vi "ICR_Finish_Sequence.vi"(8 "error in (no error)":errorcluster, 11 "QMH ICR Cluster":T1) -> (0 "error out":errorcluster, 2 "Is Finished ?":bool, 3 "QMH ICR Cluster":T1)   [LabVIEW 2024]
doc: "This VI inits a waveform generation session for both HSDIO 6541 and AWG 5421. This is a basic example that shows how to setup the board in order to generate waveforms according to a script. \n\n1. Initialize for a generation session.\n2. Assign specified channels in Channel List for dynamic operation : all = \"\" (default)\n3. Sets the Idle State for when the generation has completed : NO !!\n4. Configure the Sample clock to use the onboard clock, and configure the clock rate.\n5. Set generation mode to Scripted.\n6. Configure the Script Trigger : change to Digital Edge if waiting for an external\n trigger, and link Rising Edge and source trigger commands.\n Use PFI0 with SMB wired to the board, or any PFIxx if connected to accessory."
uses:
  controls/QMH_ICR_Cluster.ctl
  controls/HARDWARE_Resources.ctl
  controls/PROCESSING_Inputs.ctl
  controls/LOOPS_Inputs.ctl
  controls/OPO_Inputs.ctl
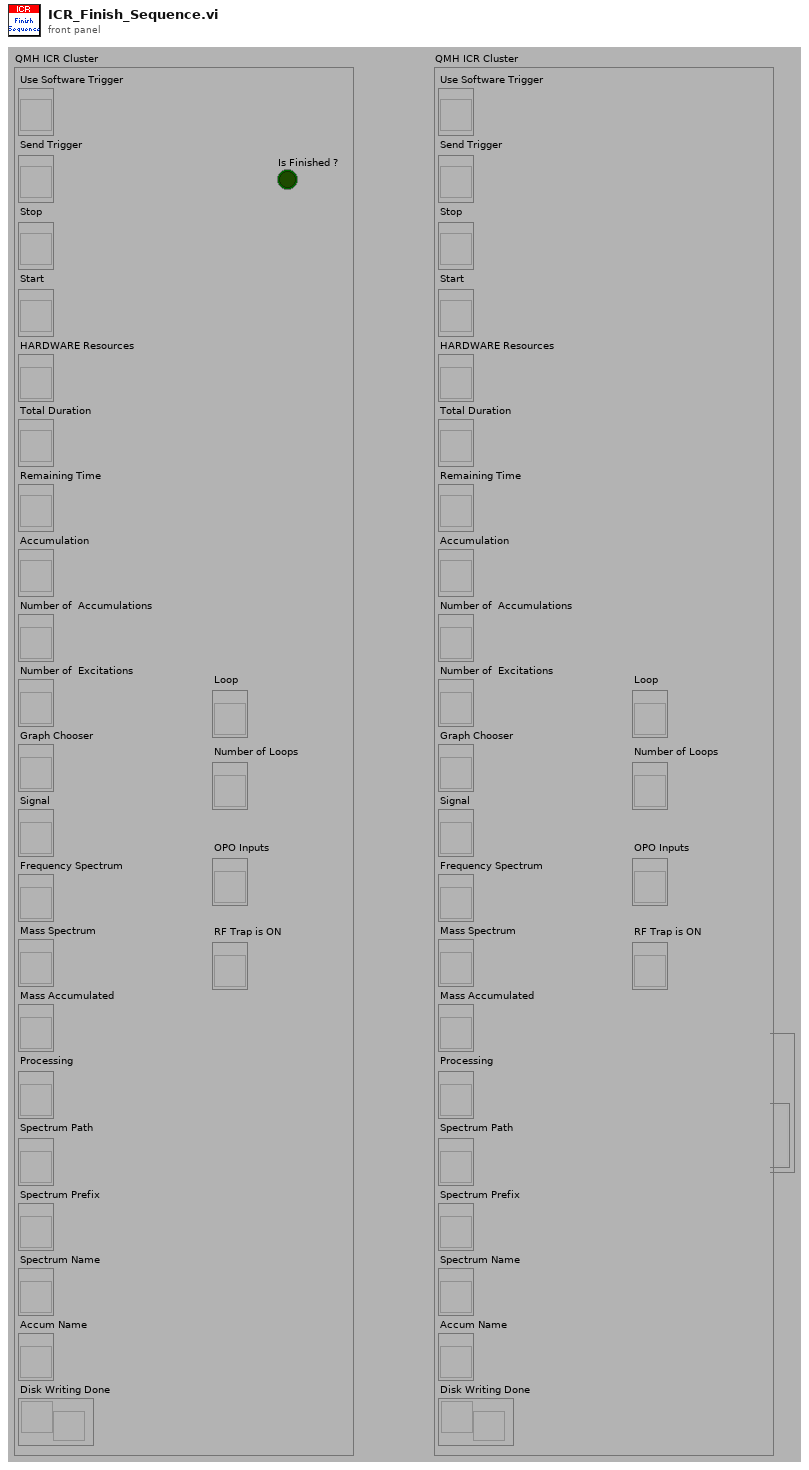
[diagram p1: front panel]
types:
  T1 = typedef "QMH_ICR_Cluster.ctl" = cluster{"Use Software Trigger":refnum<vi>, "Send Trigger":refnum<vi>, "Stop":refnum<vi>, "Start":refnum<vi>, "HARDWARE Resources":refnum<vi>, "Total Duration":refnum<vi>, "Remaining Time":refnum<vi>, "Accumulation":refnum<vi>, "Number of  Accumulations":refnum<vi>, "Number of  Excitations":refnum<vi>, "Graph Chooser":refnum<vi>, "Signal":refnum<vi>, "Frequency Spectrum":refnum<vi>, "Mass Spectrum":refnum<vi>, "Mass Accumulated":refnum<vi>, "Processing":refnum<vi>, "Spectrum Path":refnum<vi>, "Spectrum Prefix":refnum<vi>, "Spectrum Name":refnum<vi>, "Accum Name":refnum<vi>, "Disk Writing Done":refnum<notifier>, "Loop":refnum<vi>, "Number of Loops":refnum<vi>, "OPO Inputs":refnum<vi>, "RF Trap is ON":refnum<vi>}
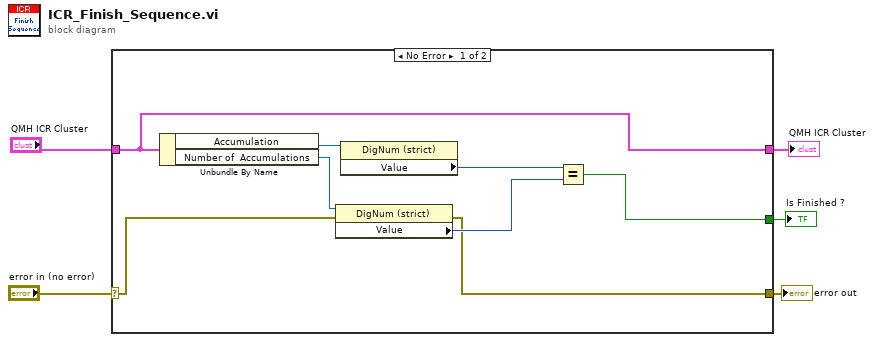
[diagram p0: block diagram]
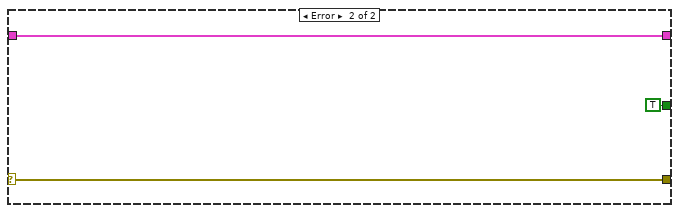
[diagram p2: hidden frame]
diagram:
  n1 = case shown="No Error" "error in (no error)" {
    selector: "error in (no error)" -> [w8 w16]
    tunnel: [w7 w16] -> w5
    tunnel: "QMH ICR Cluster" -> [w6 w15]
    tunnel: [w6 w15] -> w2
    tunnel: [w9 TRUE] -> w1
    frame No Error {
      n2 = Unbundle By Name(w6) -> ("Accumulation"=w12:refnum<vi>, "Number of  Accumulations"=w13:refnum<vi>)
      n3 = property class="DigNum (strict)"(reference=w13, error in=w8) -> (error out=w7:errorcluster, "Value"=w10:i16)  [unwired: 1 out]
      n4 = property class="DigNum (strict)"(reference=w12) -> ("Value"=w11:i16)  [unwired: 1 in, 2 out]
      n5 = Equal?(x=w11, y=w10) -> (x = y?=w9:bool)
    }
    frame Error {
    }
  }
  "error out" <- w5
  "QMH ICR Cluster" <- w2
  "Is Finished ?" <- w1
